vi "OPC Tester.vi"() -> ()   [LabVIEW 2013]
uses:
  Typedef/comm_variable_definition.ctl
  Typedef/Comm_mode_and_address_type.ctl
  Typedef/Comm_mode_type_combo.ctl
  Controls/Request Array.ctl
  Controls/All Rows Control.ctl
  Controls/OPC Data Output.ctl
panel:
  in  "Send Parameters":bool
  out "Requested Parameters":string[](array[string])
  in  "stop":bool
  in  "DeviceNet":cluster{"Buttons":bool[], "Strings":string[]}={"Buttons"=[FALSE, FALSE, FALSE, FALSE, FALSE, FALSE, FALSE, FALSE, FALSE, FALSE, FALSE, FALSE, FALSE, FALSE, FALSE, FALSE, FALSE, FALSE, FALSE, FALSE, FALSE, FALSE], "Strings"=[]}
  in  "Fieldbus":cluster{"Buttons":bool[], "Strings":string[]}={"Buttons"=[FALSE, FALSE, FALSE, FALSE, FALSE, FALSE, FALSE, FALSE, FALSE, FALSE, FALSE, FALSE, FALSE, FALSE, FALSE, FALSE, FALSE, FALSE, FALSE, FALSE, FALSE, FALSE], "Strings"=[]}
  in  "Profibus DP":cluster{"Buttons":bool[], "Strings":string[]}={"Buttons"=[FALSE, FALSE, FALSE, FALSE, FALSE, FALSE, FALSE, FALSE, FALSE, FALSE, FALSE, FALSE, FALSE, FALSE, FALSE, FALSE, FALSE, FALSE, FALSE, FALSE, FALSE, FALSE], "Strings"=[]}
  in  "Profibus PA":cluster{"Buttons":bool[], "Strings":string[]}={"Buttons"=[FALSE, FALSE, FALSE, FALSE, FALSE, FALSE, FALSE, FALSE, FALSE, FALSE, FALSE, FALSE, FALSE, FALSE, FALSE, FALSE, FALSE, FALSE, FALSE, FALSE, FALSE, FALSE], "Strings"=[]}
  in  "MODBUS":cluster{"Buttons":bool[], "Strings":string[]}={"Buttons"=[FALSE, FALSE, FALSE, FALSE, FALSE, FALSE, FALSE, FALSE, FALSE, FALSE, FALSE, FALSE, FALSE, FALSE, FALSE, FALSE, FALSE, FALSE, FALSE, FALSE, FALSE, FALSE], "Strings"=[]}
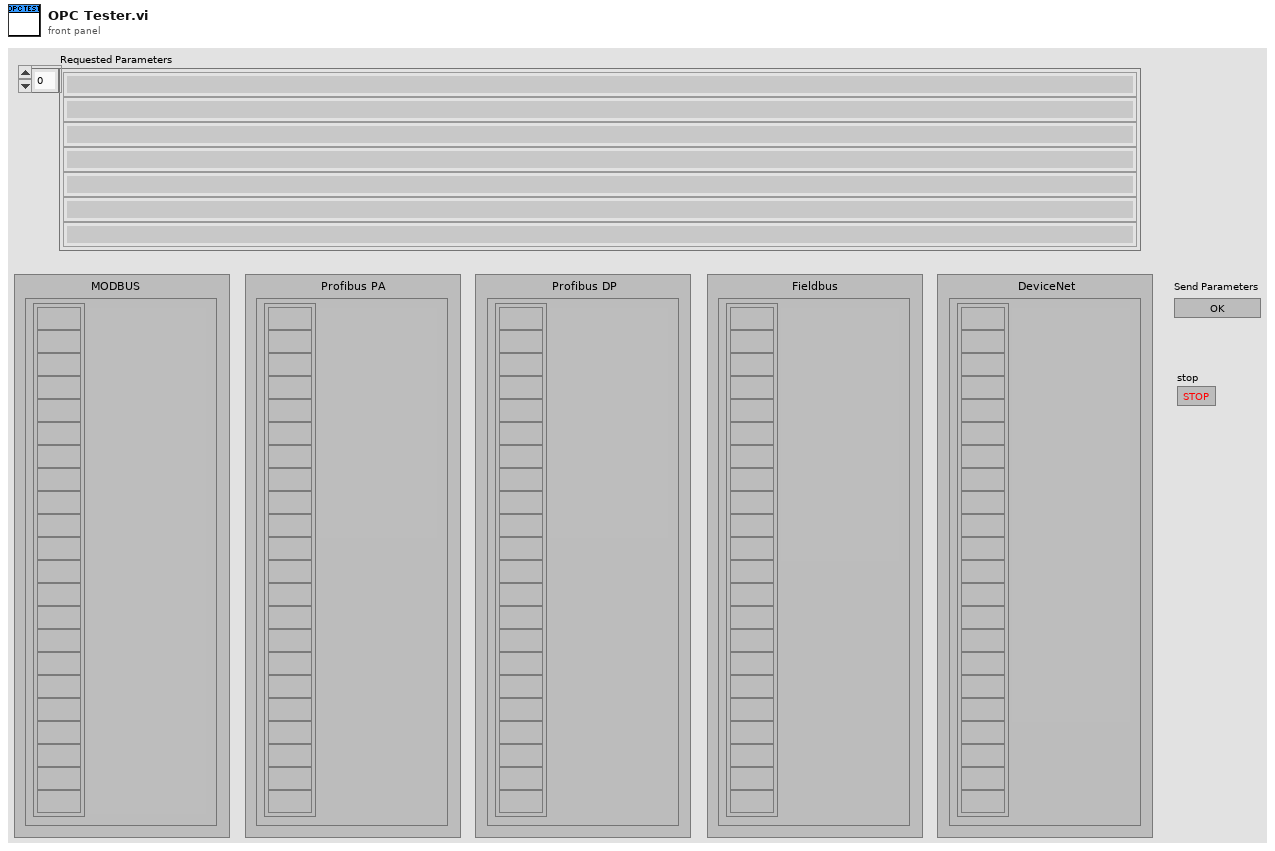
[diagram p1: front panel]
types:
  T1 = typedef "Request Array.ctl" = T2[]
  T2 = typedef "comm_variable_definition.ctl" = cluster{"General Parameter name":string, "MODBUS Register":i32, "Profibus":cluster{"Friendly name":string, "PA":cluster{"Slot":i32, "Index":i32}, "DP":cluster{"Slot":i32, "Index":i32}, "Tag":string}, "Fieldbus":cluster{"Parameter name":string, "Fieldbus Block":string, "Fieldbus Tag":string}, "data type":enum16{"float", "enum"}, "DeviceNET":cluster{"ClassId":u16, "InstanceId":u16, "AttributeId":u8}, "Cluster":T3}
  T3 = typedef "Comm_mode_and_address_type.ctl" = cluster{"address":i32, "Mode":T4}
  T4 = typedef "Comm_mode_type_combo.ctl" = u16
  T5 = typedef "All Rows Control.ctl" = string[][]
  T6 = cluster{"MODBUS":cluster{"Parameter":string, "MODBUS Register":string}[], "PA":cluster{"Parameter":string, "Profibus/Fbus Friendly Name":string, "Profibus Tag":string, "Profibus PA Slot":string, "Profibus PA Index":string}[], "DP":cluster{"Parameter":string, "Profibus/Fbus Friendly Name":string, "Profibus Tag":string, "Profibus DP Slot":string, "Profibus DP Index":string}[], "Fieldbus":cluster{"Parameter":string, "Fieldbus Friendly Name":string, "Fieldbus Block Name":string, "Fieldbus Variable":string}[], "DNET":cluster{"Parameter":string, "DNET.Class":string, "DNET.Instance":string, "DNET.Attribute":string}[]}
  T7 = cluster{"Parameter":string, "MODBUS Register":string}[]
  T8 = cluster{"Parameter":string, "Profibus/Fbus Friendly Name":string, "Profibus Tag":string, "Profibus PA Slot":string, "Profibus PA Index":string}[]
  T9 = cluster{"Parameter":string, "Profibus/Fbus Friendly Name":string, "Profibus Tag":string, "Profibus DP Slot":string, "Profibus DP Index":string}[]
  T10 = cluster{"Parameter":string, "Fieldbus Friendly Name":string, "Fieldbus Block Name":string, "Fieldbus Variable":string}[]
  T11 = cluster{"Parameter":string, "DNET.Class":string, "DNET.Instance":string, "DNET.Attribute":string}[]
  T12 = cluster{"Buttons":refnum<vi>, "Buttons":refnum<vi>, "Buttons":refnum<vi>, "Buttons":refnum<vi>, "Buttons":refnum<vi>}
  T13 = typedef "OPC Data Output.ctl" = cluster{"Data Out Array":cluster{"error out":errorcluster, "Output":variant, "Cluster.Mode":T4, "Parameter name":string}[], "Timestamp":string, "Loop Time":dbl}
  T14 = cluster{"Parameter":string, "MODBUS Register":string}
  T15 = cluster{"Parameter":string, "Profibus/Fbus Friendly Name":string, "Profibus Tag":string, "Profibus PA Slot":string, "Profibus PA Index":string}
  T16 = cluster{"Parameter":string, "Profibus/Fbus Friendly Name":string, "Profibus Tag":string, "Profibus DP Slot":string, "Profibus DP Index":string}
  T17 = cluster{"Parameter":string, "Fieldbus Friendly Name":string, "Fieldbus Block Name":string, "Fieldbus Variable":string}
  T18 = cluster{"Parameter":string, "DNET.Class":string, "DNET.Instance":string, "DNET.Attribute":string}
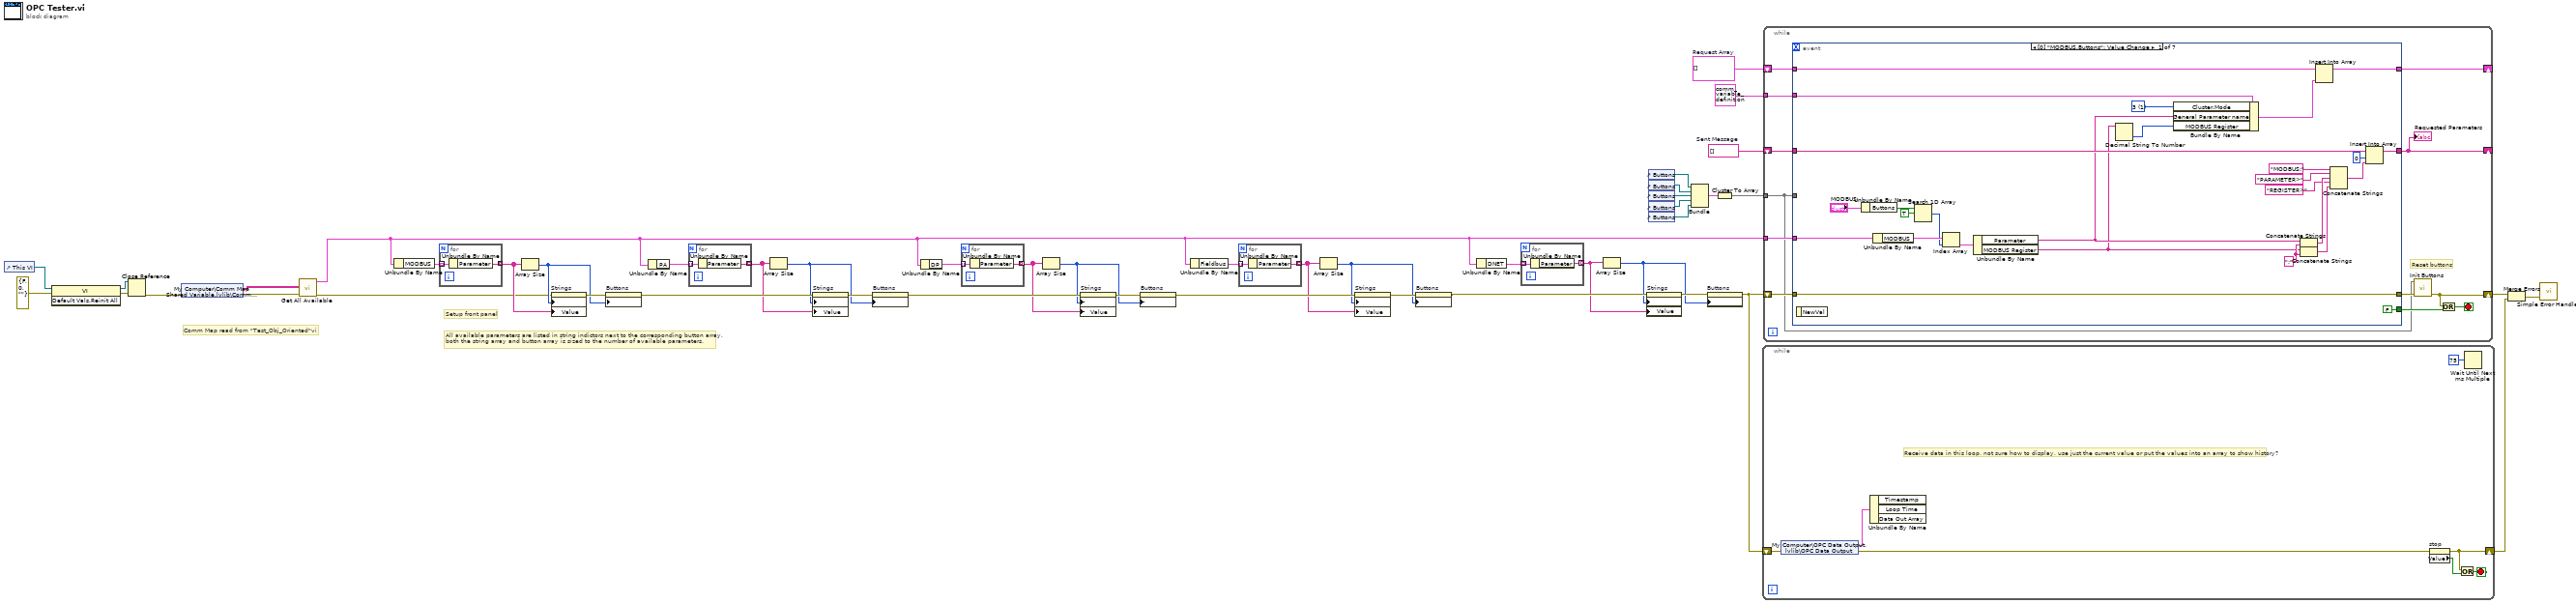
[diagram p0: block diagram]
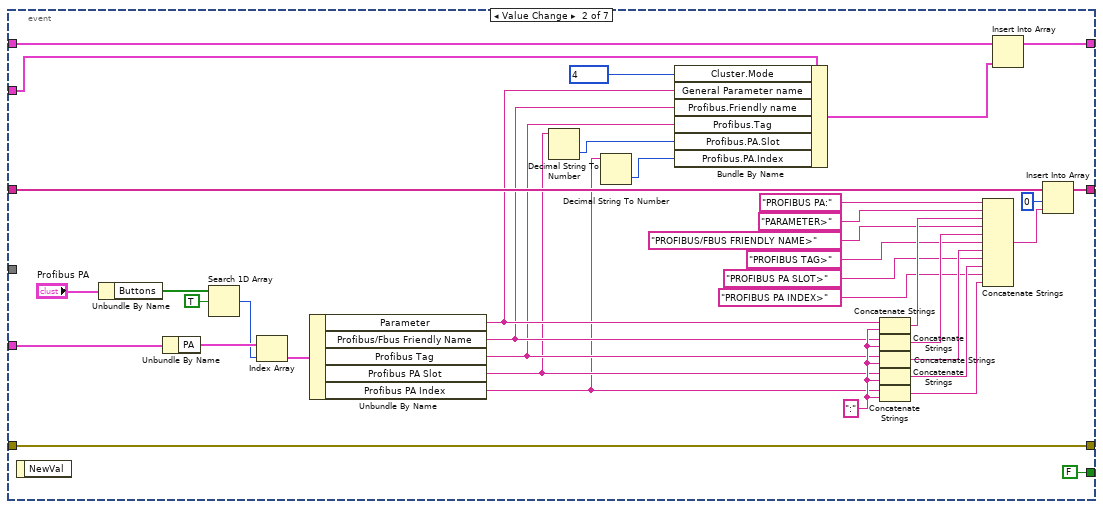
[diagram p2: hidden frame]
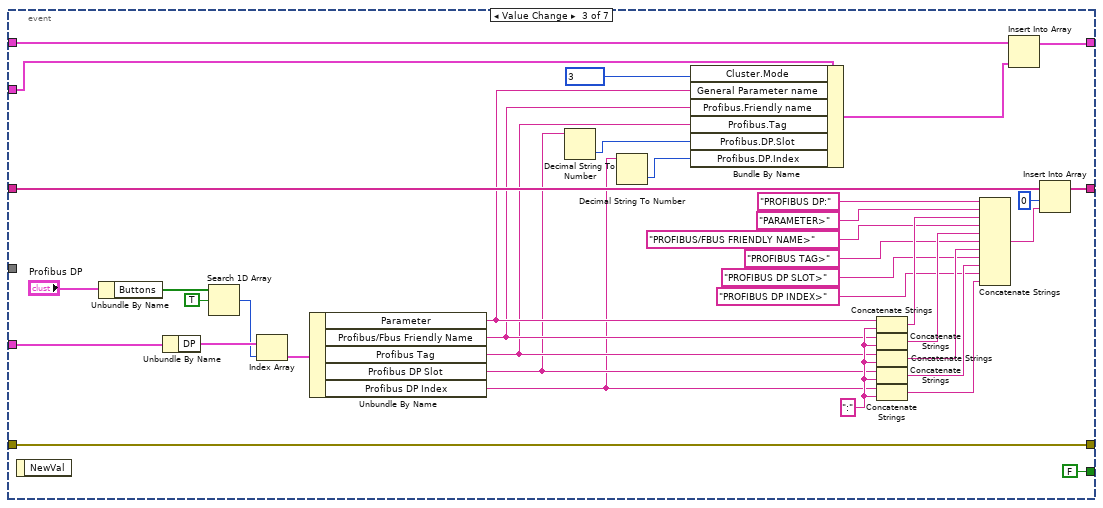
[diagram p3: hidden frame]
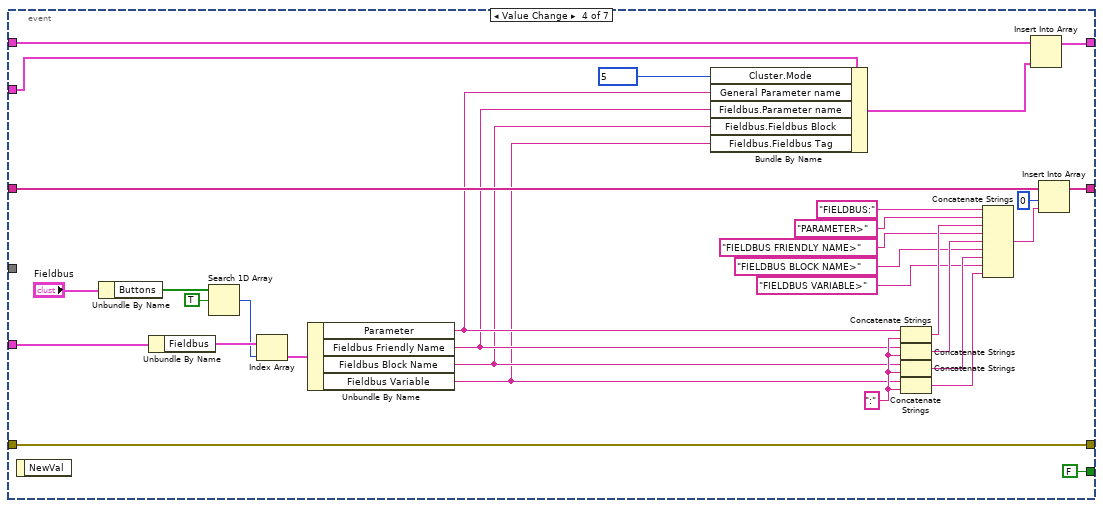
[diagram p4: hidden frame]
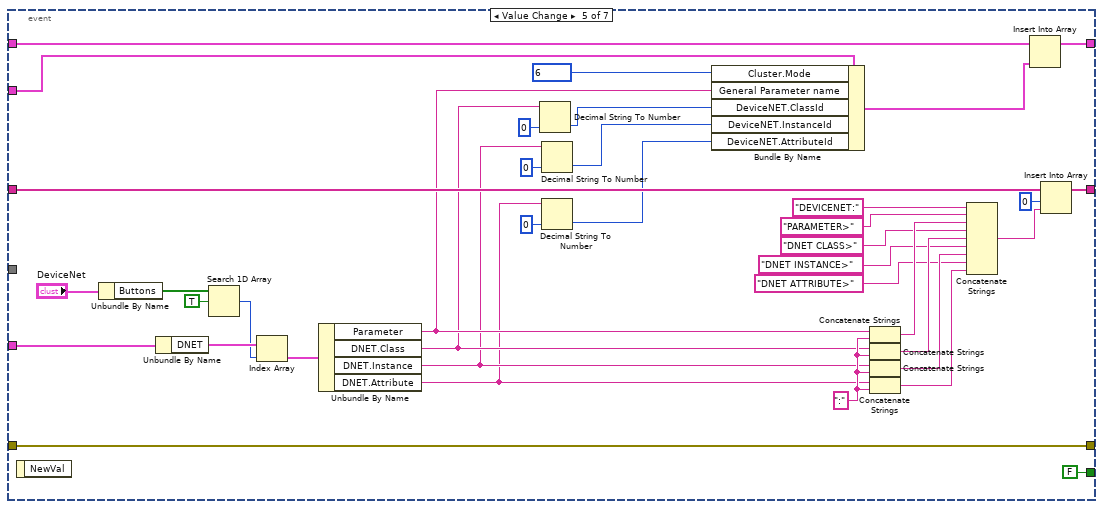
[diagram p5: hidden frame]
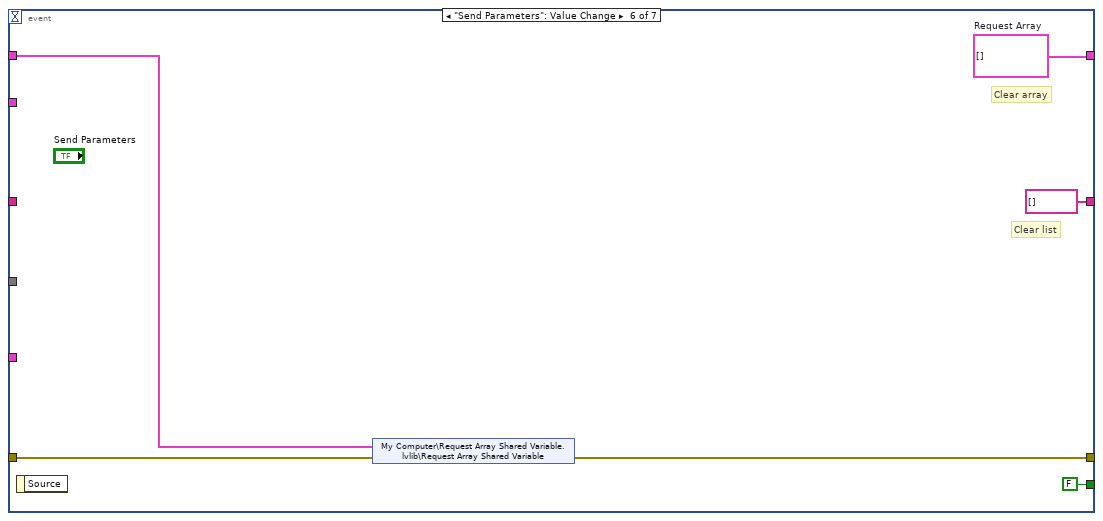
[diagram p6: hidden frame]
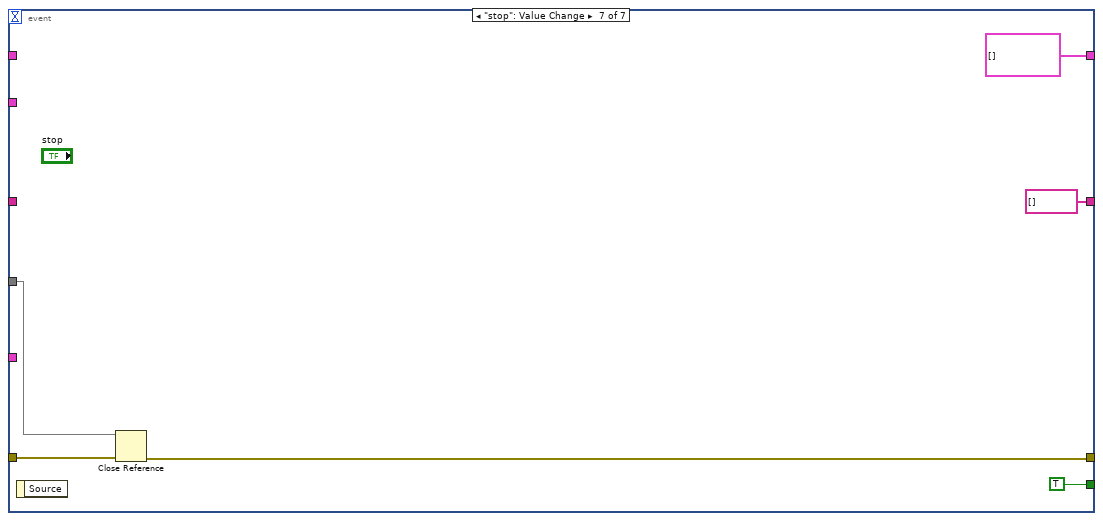
[diagram p7: hidden frame]
diagram:
  w5 = T1 []  # Request Array
  w13 = string[] []  # Sent Message
  # "Comm Map read from \"Test_Obj_Oriented\"vi"
  # "Setup front panel"
  # "All available parameters are listed in string indictors next to the corresponding button array,\nboth the string array and button array is sized to the number of available parameters."
  n1 = control-ref of="This VI"() -> (w46:refnum<vi>)
  n2 = invoke class="VI" method="Default Vals.Reinit All"(reference=w46, error in=errorcluster {"status"=FALSE, "code"=0, "source"=""} ("error constant")) -> (reference out=w43:refnum<vi>, error out=w44:errorcluster)  [unwired: 1 in, 1 out]
  n3 = Close Reference(reference=w43, error in (no error)=w44) -> (error out=w11:errorcluster)
  n4 = shared-variable "My Computer\\Comm Map Shared Variable.lvlib\\Comm Map"(error in=w11) -> (w9:T5, error out=w10:errorcluster)
  n5 = call "Get All Available.vi"("error in"=w10, "all rows"=w9) -> ("error out"=w8:errorcluster, "Available Parameters"=w12:T6)  [unwired: 8 in]
  n6 = Unbundle By Name(w12) -> ("MODBUS"=w42:T7)
  n7 = for {
    tunnel: w42 -> [w49] mode=indexing
    tunnel: [w48] -> w40 mode=indexing
    n8 = Unbundle By Name(w49) -> ("Parameter"=w48:string)
  }
  n9 = Array Size(array=w40) -> (size(s)=w39:i32)
  n10 = property on="Strings" class="Arr (strict)"(error in=w8, "Number of Rows"=w39, "Value"=w40) -> (error out=w41:errorcluster)  [unwired: 1 in, 1 out]
  n11 = property on="Buttons" class="Arr"(error in=w41, "Number of Rows"=w39) -> (error out=w36:errorcluster)  [unwired: 1 in, 1 out]
  n12 = Unbundle By Name(w12) -> ("PA"=w38:T8)
  n13 = for {
    tunnel: w38 -> [w51] mode=indexing
    tunnel: [w50] -> w35 mode=indexing
    n14 = Unbundle By Name(w51) -> ("Parameter"=w50:string)
  }
  n15 = Array Size(array=w35) -> (size(s)=w34:i32)
  n16 = property on="Strings" class="Arr (strict)"(error in=w36, "Number of Rows"=w34, "Value"=w35) -> (error out=w37:errorcluster)  [unwired: 1 in, 1 out]
  n17 = property on="Buttons" class="Arr"(error in=w37, "Number of Rows"=w34) -> (error out=w31:errorcluster)  [unwired: 1 in, 1 out]
  n18 = Unbundle By Name(w12) -> ("DP"=w33:T9)
  n19 = for {
    tunnel: w33 -> [w53] mode=indexing
    tunnel: [w52] -> w30 mode=indexing
    n20 = Unbundle By Name(w53) -> ("Parameter"=w52:string)
  }
  n21 = Array Size(array=w30) -> (size(s)=w29:i32)
  n22 = property on="Strings" class="Arr (strict)"(error in=w31, "Number of Rows"=w29, "Value"=w30) -> (error out=w32:errorcluster)  [unwired: 1 in, 1 out]
  n23 = property on="Buttons" class="Arr"(error in=w32, "Number of Rows"=w29) -> (error out=w47:errorcluster)  [unwired: 1 in, 1 out]
  n24 = Unbundle By Name(w12) -> ("Fieldbus"=w28:T10)
  n25 = for {
    tunnel: w28 -> [w55] mode=indexing
    tunnel: [w54] -> w27 mode=indexing
    n26 = Unbundle By Name(w55) -> ("Parameter"=w54:string)
  }
  n27 = Array Size(array=w27) -> (size(s)=w25:i32)
  n28 = property on="Strings" class="Arr (strict)"(error in=w47, "Number of Rows"=w25, "Value"=w27) -> (error out=w26:errorcluster)  [unwired: 1 in, 1 out]
  n29 = property on="Buttons" class="Arr"(error in=w26, "Number of Rows"=w25) -> (error out=w22:errorcluster)  [unwired: 1 in, 1 out]
  n30 = Unbundle By Name(w12) -> ("DNET"=w24:T11)
  n31 = for {
    tunnel: w24 -> [w57] mode=indexing
    tunnel: [w56] -> w21 mode=indexing
    n32 = Unbundle By Name(w57) -> ("Parameter"=w56:string)
  }
  n33 = Array Size(array=w21) -> (size(s)=w20:i32)
  n34 = property on="Strings" class="Arr (strict)"(error in=w22, "Number of Rows"=w20, "Value"=w21) -> (error out=w23:errorcluster)  [unwired: 1 in, 1 out]
  n35 = control-ref of="Buttons"() -> (w14:refnum<vi>)
  n36 = control-ref of="Buttons"() -> (w15:refnum<vi>)
  n37 = control-ref of="Buttons"() -> (w16:refnum<vi>)
  n38 = control-ref of="Buttons"() -> (w17:refnum<vi>)
  n39 = control-ref of="Buttons"() -> (w18:refnum<vi>)
  n40 = Bundle("Buttons"=w14, "Buttons"=w15, "Buttons"=w16, "Buttons"=w17, "Buttons"=w18) -> (w19:T12)  [unwired: 1 in]
  n41 = property on="Buttons" class="Arr"(error in=w23, "Number of Rows"=w20) -> (error out=w4:errorcluster)  [unwired: 1 in, 1 out]
  n42 = Cluster To Array(cluster=w19) -> (array=w6:refnum<vi>[])
  n43 = while {
    shift-right: [w61] -> w1
    shift-left: w4 -> [w63]
    stop <- w60 stop-if-true
    # "Receive data in this loop, not sure how to display, use just the current value or put the values into an array to show history?"
    n44 = shared-variable "My Computer\\OPC Data Output.lvlib\\OPC Data Output"(error in=w63) -> (w59:T13, error out=w58:errorcluster)
    n45 = Unbundle By Name(w59) -> ()  [unwired: 3 out]
    n46 = property on="stop" class="Bool (strict)"(error in=w58) -> (error out=w61:errorcluster, "Value"=w62:bool)  [unwired: 1 in, 1 out]
    n47 = Or(x=w61, y=w62) -> (x .or. y?=w60:bool)
    n48 = Wait Until Next ms Multiple(millisecond multiple=u32 75) -> ()  [unwired: 1 out]
  }
  n49 = while {
    tunnel: w12 -> [w76]
    shift-right: [w72] -> _
    shift-left: w13 -> [w75]
    shift-right: [w66] -> w2
    shift-left: w4 -> [w73]
    tunnel: T2 {"General Parameter name"="", "MODBUS Register"=0, "Profibus"={"Friendly name"="", "PA"={"Slot"=0, "Index"=0}, "DP"={"Slot"=0, "Index"=0}, "Tag"=""}, "Fieldbus"={"Parameter name"="", "Fieldbus Block"="", "Fieldbus Tag"=""}, "data type"=enum."float", "DeviceNET"={"ClassId"=0, "InstanceId"=0, "AttributeId"=0}, "Cluster"={"address"=0, "Mode"=0}} ("Comm definition type") -> [w71]
    shift-right: [w69] -> _
    shift-left: w5 -> [w70]
    tunnel: w6 -> [w65]
    stop <- w74 stop-if-true
    # "Reset buttons"
    n50 = event shown="[0] \"MODBUS.Buttons\": Value Change" {
      selector: _ -> [_ _ _ _ _ _ _]
      dyn-events: _ -> [_ _ _ _ _ _ _]
      timeout: _ -> [_ _ _ _ _ _ _]
      tunnel: w73 -> [w96 w134 w171 w203 w241 w250 w257]
      tunnel: w76 -> [w100 w138 w175 w207 w245 _ _]
      tunnel: [w96 w134 w171 w203 w241 w249 w255] -> w67
      tunnel: [w94 w132 w169 w201 w239 string[] [] ("Sent Message") string[] [] ("Sent Message")] -> w72
      tunnel: w75 -> [w95 w133 w170 w202 w240 _ _]
      tunnel: w71 -> [w85 w113 w145 w184 w221 _ _]
      tunnel: w70 -> [w81 w114 w149 w185 w223 w248 _]
      tunnel: [w80 w105 w148 w179 w222 w251 T2[] [] ("Array of comm typedef")] -> w69
      tunnel: [FALSE FALSE FALSE FALSE FALSE FALSE TRUE] -> w68
      tunnel: w65 -> [_ _ _ _ _ _ w256]
      event "MODBUS.Buttons": Value Change {
        w77 = T4 1 items=["Modbus-1", "3"] ("Mode")
        w87 = ":" ("string")
        n51 = event-data() -> ()  [unwired: 1 in, 1 out]
        n52 = Unbundle By Name("MODBUS") -> ("Buttons"=w102:bool[])
        n53 = Unbundle By Name(w100) -> ("MODBUS"=w99:T7)
        n54 = Search 1D Array(1D array=w102, element=TRUE) -> (index of element=w98:i32)  [unwired: 1 in]
        n55 = Index Array(array=w99, index=w98) -> (element=w97:T14)
        n56 = Unbundle By Name(w97) -> ("Parameter"=w84:string, "MODBUS Register"=w83:string)
        n57 = Decimal String To Number(string=w83) -> (number=w82:i32)  [unwired: 2 in, 1 out]
        n58 = Bundle By Name(cluster=w85, "Cluster.Mode"=w77, "General Parameter name"=w84, "MODBUS Register"=w82) -> (w79:T2)
        n59 = Concatenate Strings(w84, w87) -> (w90:string)
        n60 = Concatenate Strings(w83, w87) -> (w88:string)
        n61 = Insert Into Array(array=w81, new element=w79) -> (w80:T1)  [unwired: 1 in]
        n62 = Concatenate Strings("MODBUS:" ("string"), "PARAMETER>" ("string"), w90, "REGISTER>" ("string"), w88) -> (w91:string)
        n63 = Insert Into Array(array=w95, index=0, new element=w91) -> (w94:string[])
      }
      event "Profibus PA.Buttons": Value Change {
        w104 = T4 4 items=["Modbus-1", "3"] ("Mode")
        w128 = ":" ("string")
        n64 = event-data() -> ()  [unwired: 1 in, 1 out]
        n65 = Unbundle By Name("Profibus PA") -> ("Buttons"=w140:bool[])
        n66 = Unbundle By Name(w138) -> ("PA"=w137:T8)
        n67 = Search 1D Array(1D array=w140, element=TRUE) -> (index of element=w136:i32)  [unwired: 1 in]
        n68 = Index Array(array=w137, index=w136) -> (element=w135:T15)
        n69 = Unbundle By Name(w135) -> ("Parameter"=w112:string, "Profibus/Fbus Friendly Name"=w111:string, "Profibus Tag"=w110:string, "Profibus PA Slot"=w109:string, "Profibus PA Index"=w107:string)
        n70 = Decimal String To Number(string=w109) -> (number=w108:i32)  [unwired: 2 in, 1 out]
        n71 = Decimal String To Number(string=w107) -> (number=w106:i32)  [unwired: 2 in, 1 out]
        n72 = Bundle By Name(cluster=w113, "Cluster.Mode"=w104, "General Parameter name"=w112, "Profibus.Friendly name"=w111, "Profibus.Tag"=w110, "Profibus.PA.Slot"=w108, "Profibus.PA.Index"=w106) -> (w115:T2)
        n73 = Concatenate Strings(w112, w128) -> (w127:string)
        n74 = Concatenate Strings(w111, w128) -> (w125:string)
        n75 = Concatenate Strings(w110, w128) -> (w123:string)
        n76 = Concatenate Strings(w109, w128) -> (w121:string)
        n77 = Concatenate Strings(w107, w128) -> (w119:string)
        n78 = Concatenate Strings("PROFIBUS PA:" ("string"), "PARAMETER>" ("string"), w127, "PROFIBUS/FBUS FRIENDLY NAME>" ("string"), w125, "PROFIBUS TAG>" ("string"), w123, "PROFIBUS PA SLOT>" ("string"), w121, "PROFIBUS PA INDEX>" ("string"), w119) -> (w118:string)
        n79 = Insert Into Array(array=w114, new element=w115) -> (w105:T1)  [unwired: 1 in]
        n80 = Insert Into Array(array=w133, index=0, new element=w118) -> (w132:string[])
      }
      event "Profibus DP.Buttons": Value Change {
        w141 = T4 3 items=["Modbus-1", "3"] ("Mode")
        w166 = ":" ("string")
        n81 = event-data() -> ()  [unwired: 1 in, 1 out]
        n82 = Unbundle By Name("Profibus DP") -> ("Buttons"=w177:bool[])
        n83 = Unbundle By Name(w175) -> ("DP"=w174:T9)
        n84 = Search 1D Array(1D array=w177, element=TRUE) -> (index of element=w173:i32)  [unwired: 1 in]
        n85 = Index Array(array=w174, index=w173) -> (element=w172:T16)
        n86 = Unbundle By Name(w172) -> ("Parameter"=w147:string, "Profibus/Fbus Friendly Name"=w146:string, "Profibus Tag"=w144:string, "Profibus DP Slot"=w143:string, "Profibus DP Index"=w142:string)
        n87 = Decimal String To Number(string=w143) -> (number=w151:i32)  [unwired: 2 in, 1 out]
        n88 = Decimal String To Number(string=w142) -> (number=w150:i32)  [unwired: 2 in, 1 out]
        n89 = Bundle By Name(cluster=w145, "Cluster.Mode"=w141, "General Parameter name"=w147, "Profibus.Friendly name"=w146, "Profibus.Tag"=w144, "Profibus.DP.Slot"=w151, "Profibus.DP.Index"=w150) -> (w152:T2)
        n90 = Concatenate Strings(w147, w166) -> (w165:string)
        n91 = Concatenate Strings(w146, w166) -> (w163:string)
        n92 = Concatenate Strings(w144, w166) -> (w161:string)
        n93 = Concatenate Strings(w143, w166) -> (w159:string)
        n94 = Concatenate Strings(w142, w166) -> (w157:string)
        n95 = Concatenate Strings("PROFIBUS DP:" ("string"), "PARAMETER>" ("string"), w165, "PROFIBUS/FBUS FRIENDLY NAME>" ("string"), w163, "PROFIBUS TAG>" ("string"), w161, "PROFIBUS DP SLOT>" ("string"), w159, "PROFIBUS DP INDEX>" ("string"), w157) -> (w156:string)
        n96 = Insert Into Array(array=w149, new element=w152) -> (w148:T1)  [unwired: 1 in]
        n97 = Insert Into Array(array=w170, index=0, new element=w156) -> (w169:string[])
      }
      event "Fieldbus.Buttons": Value Change {
        w178 = T4 5 items=["Modbus-1", "3"] ("Mode")
        w199 = ":" ("string")
        n98 = event-data() -> ()  [unwired: 1 in, 1 out]
        n99 = Unbundle By Name("Fieldbus") -> ("Buttons"=w209:bool[])
        n100 = Unbundle By Name(w207) -> ("Fieldbus"=w206:T10)
        n101 = Search 1D Array(1D array=w209, element=TRUE) -> (index of element=w205:i32)  [unwired: 1 in]
        n102 = Index Array(array=w206, index=w205) -> (element=w204:T17)
        n103 = Unbundle By Name(w204) -> ("Parameter"=w183:string, "Fieldbus Friendly Name"=w182:string, "Fieldbus Block Name"=w181:string, "Fieldbus Variable"=w180:string)
        n104 = Bundle By Name(cluster=w184, "Cluster.Mode"=w178, "General Parameter name"=w183, "Fieldbus.Parameter name"=w182, "Fieldbus.Fieldbus Block"=w181, "Fieldbus.Fieldbus Tag"=w180) -> (w186:T2)
        n105 = Concatenate Strings(w183, w199) -> (w195:string)
        n106 = Concatenate Strings(w182, w199) -> (w193:string)
        n107 = Concatenate Strings(w181, w199) -> (w191:string)
        n108 = Concatenate Strings(w180, w199) -> (w189:string)
        n109 = Concatenate Strings("FIELDBUS:" ("string"), "PARAMETER>" ("string"), w195, "FIELDBUS FRIENDLY NAME>" ("string"), w193, "FIELDBUS BLOCK NAME>" ("string"), w191, "FIELDBUS VARIABLE>" ("string"), w189) -> (w198:string)
        n110 = Insert Into Array(array=w185, new element=w186) -> (w179:T1)  [unwired: 1 in]
        n111 = Insert Into Array(array=w202, index=0, new element=w198) -> (w201:string[])
      }
      event "DeviceNet.Buttons": Value Change {
        w210 = T4 6 items=["Modbus-1", "3"] ("Mode")
        w237 = ":" ("string")
        n112 = event-data() -> ()  [unwired: 1 in, 1 out]
        n113 = Unbundle By Name("DeviceNet") -> ("Buttons"=w247:bool[])
        n114 = Unbundle By Name(w245) -> ("DNET"=w244:T11)
        n115 = Search 1D Array(1D array=w247, element=TRUE) -> (index of element=w243:i32)  [unwired: 1 in]
        n116 = Index Array(array=w244, index=w243) -> (element=w242:T18)
        n117 = Unbundle By Name(w242) -> ("Parameter"=w220:string, "DNET.Class"=w219:string, "DNET.Instance"=w216:string, "DNET.Attribute"=w214:string)
        n118 = Decimal String To Number(string=w219, default (0L)=u16 0 ("default (0 I32)")) -> (number=w213:u16)  [unwired: 1 in, 1 out]
        n119 = Decimal String To Number(string=w216, default (0L)=u16 0 ("default (0 I32)")) -> (number=w212:u16)  [unwired: 1 in, 1 out]
        n120 = Decimal String To Number(string=w214, default (0L)=u8 0 ("default (0 I32)")) -> (number=w211:u8)  [unwired: 1 in, 1 out]
        n121 = Bundle By Name(cluster=w221, "Cluster.Mode"=w210, "General Parameter name"=w220, "DeviceNET.ClassId"=w213, "DeviceNET.InstanceId"=w212, "DeviceNET.AttributeId"=w211) -> (w224:T2)
        n122 = Concatenate Strings(w220, w237) -> (w234:string)
        n123 = Concatenate Strings(w219, w237) -> (w232:string)
        n124 = Concatenate Strings(w216, w237) -> (w230:string)
        n125 = Concatenate Strings(w214, w237) -> (w228:string)
        n126 = Concatenate Strings("DEVICENET:" ("string"), "PARAMETER>" ("string"), w234, "DNET CLASS>" ("string"), w232, "DNET INSTANCE>" ("string"), w230, "DNET ATTRIBUTE>" ("string"), w228) -> (w227:string)
        n127 = Insert Into Array(array=w223, new element=w224) -> (w222:T1)  [unwired: 1 in]
        n128 = Insert Into Array(array=w240, index=0, new element=w227) -> (w239:string[])
      }
      event "Send Parameters": Value Change {
        w251 = T1 []  # Request Array
        # "Clear list"
        # "Clear array"
        n129 = event-data() -> ()  [unwired: 1 in, 1 out]
        n130 = shared-variable "My Computer\\Request Array Shared Variable.lvlib\\Request Array Shared Variable"(w248, error in=w250) -> (error out=w249:errorcluster)
      }
      event "stop": Value Change {
        n131 = event-data() -> ()  [unwired: 1 in, 1 out]
        n132 = Close Reference(reference=w256, error in (no error)=w257) -> (error out=w255:errorcluster)
      }
    }
    "Requested Parameters" <- w72
    n133 = call "Init Buttons.vi"("error in (no error)"=w67, "Refs In"=w65) -> ("error out"=w66:errorcluster)  [unwired: 9 in]
    n134 = Or(x=w66, y=w68) -> (x .or. y?=w74:bool)
  }
  n135 = Merge Errors(w2, w1) -> (w3:errorcluster)
  n136 = call <vilib>:"Simple Error Handler.vi"("error in (no error)"=w3) -> ()  [unwired: 4 in, 5 out]
